vi "load, hough.vi"() -> ()   [LabVIEW 2011]
uses:
  <userlib>/labvvis/Many Hough Lines.ctl
  <userlib>/labvvis/Hough Line.ctl
  <userlib>/labvvis/New Image/New Image (Grey).vi
  <userlib>/labvvis/labvvis.lvlib
panel:
  out "Total Number of Lines":u16
  out "Output Lines":T1
  out "Error":string
  in  "path to JPEG file":path
  out "new picture":picture
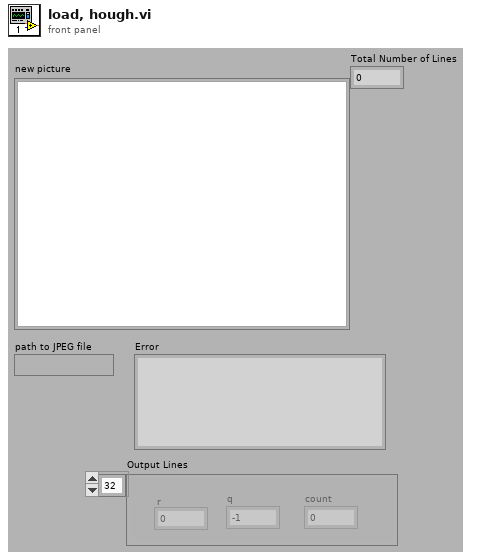
[diagram p1: front panel]
types:
  T1 = typedef "labvvis.lvlib/Many Hough Lines.ctl" = T2[]
  T2 = typedef "labvvis.lvlib/Hough Line.ctl" = cluster{"r":dbl, "q":i16, "count":i16}
  T3 = typedef "imagedata.ctl" = cluster{"image type":i32, "image depth":i32, "image":u8[], "mask":u8[], "colors":u32[], "Rectangle":cluster{"left":i16, "top":i16, "right":i16, "bottom":i16}}
  T4 = typedef "labvvis.lvlib/VVIS Image.ctl" = cluster{"Image ID":i16, "Channel ID":i16}
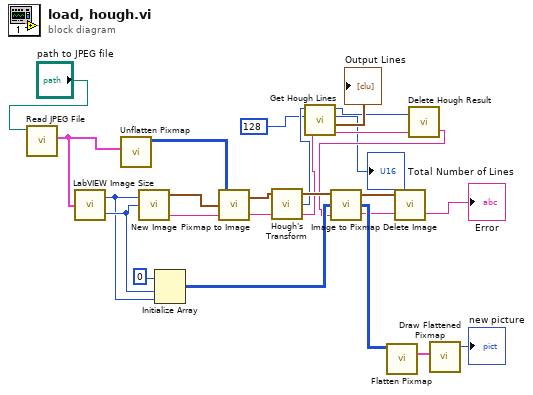
[diagram p0: block diagram]
diagram:
  n1 = call <vilib>:"Read JPEG File.vi"("path to JPEG file"="path to JPEG file") -> ("image data"=w14:T3)  [unwired: 8 in, 2 out]
  n2 = call <userlib>:"LabVIEW Image Size.vi"("Cluster"=w14) -> ("Width"=w12:i16, "Height"=w13:i16)
  n3 = call <vilib>:"Unflatten Pixmap.vi"("image data"=w14) -> ("24-bit pixmap"=w21:u32[][])  [unwired: 4 in, 6 out]
  n4 = call-poly <userlib>:"New Image.vi"("Height"=w13, "Width"=w12) -> ("Error"=w15:string, "VVIS Image"=w22:T4)  [unwired: 2 in]
  n5 = Initialize Array(0, w13, w12) -> (w19:i32[][])
  n6 = call <userlib>:"Pixmap to Image.vi"("Error"=w15, "Output Image"=w22, "Input Pixmap"=w21) -> ("Error"=w4:string, "Output Image"=w11:T4)
  n7 = call <userlib>:"Hough's Transform.vi"("Error"=w4, "Input Image"=w11) -> ("Error"=w6:string, "Hough's Transform's Result"=w7:i16, "Input Image"=w10:T4)  [unwired: 1 in]
  n8 = call <userlib>:"Get Hough Lines.vi"("Error"=w6, "Threshold"=i16 128, "Hough's Transform's Result"=w7) -> ("Error"=w9:string, "Output Lines"=→"Output Lines":T1, "Total Number of Lines"=→"Total Number of Lines":u16, "Hough's Transform's Result"=w2:i16)  [unwired: 1 in]
  n9 = call <userlib>:"Delete Hough Result.vi"("Error"=w9, "Hough's Transform's Result"=w2) -> ("Error"=w5:string)  [unwired: 1 out]
  n10 = call <userlib>:"Image to Pixmap.vi"("Error"=w5, "Output Pixmap"=w19, "Image"=w10) -> ("Error"=w17:string, "Output Pixmap"=w20:u32[][], "Image"=w18:T4)
  n11 = call <vilib>:"Flatten Pixmap.vi"("24-bit pixmap"=w20) -> ("image data"=w23:T3)  [unwired: 10 in]
  n12 = call <userlib>:"Delete Image.vi"("Error"=w17, "Image"=w18) -> ("Error"=→"Error":string)  [unwired: 1 in]
  n13 = call <vilib>:"Draw Flattened Pixmap.vi"("image data"=w23) -> ("new picture"=→"new picture":picture)  [unwired: 8 in]
